vi "GetPaths.vi"(11 "error in":errorcluster) -> (6 "DDMM_Factory_Paths":T1, 15 "error out":errorcluster)   [LabVIEW 2020, in "DMMFactory.lvlib" / "DMMFactory.lvclass"]
uses:
  DMMFactory.lvclass
  TypeDef/DMM_Factory_Paths.ctl
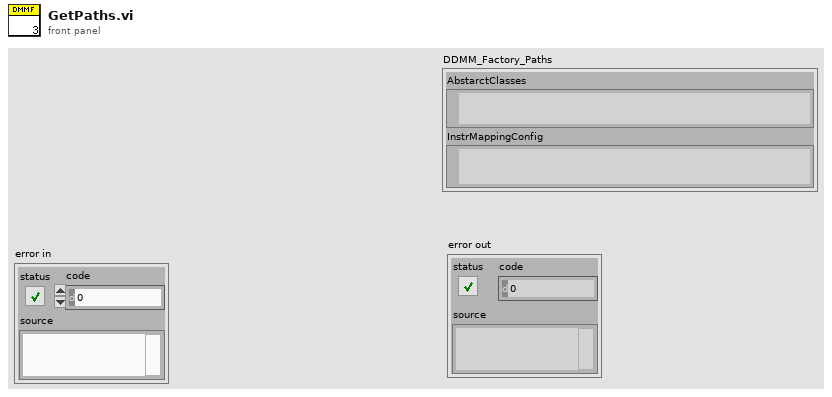
[diagram p1: front panel]
types:
  T1 = typedef "DMMFactory.lvlib/DMMFactory.lvclass/DMM_Factory_Paths.ctl" = cluster{"AbstarctClasses":path, "InstrMappingConfig":path}
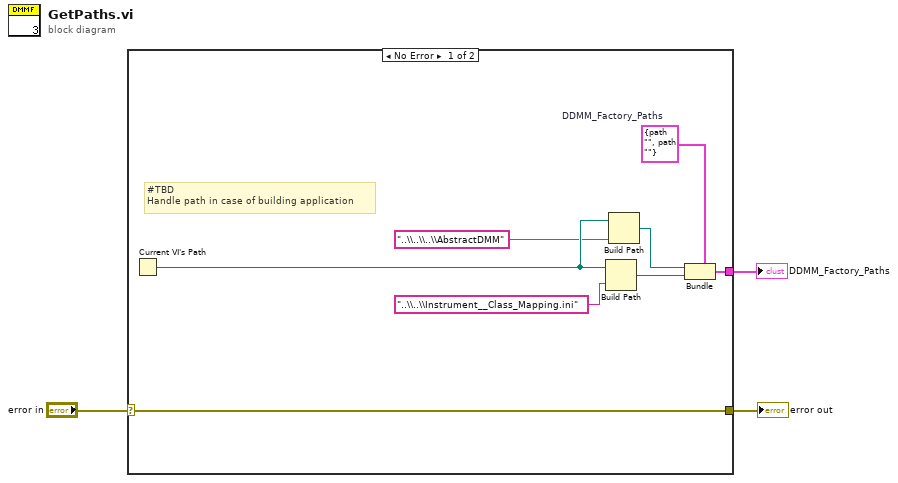
[diagram p0: block diagram]
diagram:
  n1 = case shown="No Error" "error in" {
    selector: "error in" -> [w4 w12]
    tunnel: [w5 _] -> w3
    tunnel: [w4 w12] -> w1
    frame No Error {
      w6 = T1 {"AbstarctClasses"=path "", "InstrMappingConfig"=path ""}  # DDMM_Factory_Paths
      # "#TBD\nHandle path in case of building application"
      n2 = Current VI's Path() -> (path=w9:path)
      n3 = Build Path(base path=w9, name or relative path="..\\..\\Instrument__Class_Mapping.ini") -> (appended path=w10:path)
      n4 = Build Path(base path=w9, name or relative path="..\\..\\..\\AbstractDMM") -> (appended path=w7:path)
      n5 = Bundle(cluster=w6, "AbstarctClasses"=w7, "InstrMappingConfig"=w10) -> (w5:T1)
    }
    frame Error {
    }
  }
  "error out" <- w1
  "DDMM_Factory_Paths" <- w3
